vi "GetConfig.vi"() -> (3 "mail info out":T1)   [LabVIEW 2017]
uses:
  <vilib>/Utility/config.llb/Read Key (String).vi
  <vilib>/Utility/config.llb/Read Key (I32).vi
  <vilib>/Utility/config.llb/NI_LVConfig.lvlib
panel:
  in  "mail info":T1={"host"="smtp-mail.outlook.com", "port"=587, "username"="", "password"="", "From"="", "to"="", "subject"=""}
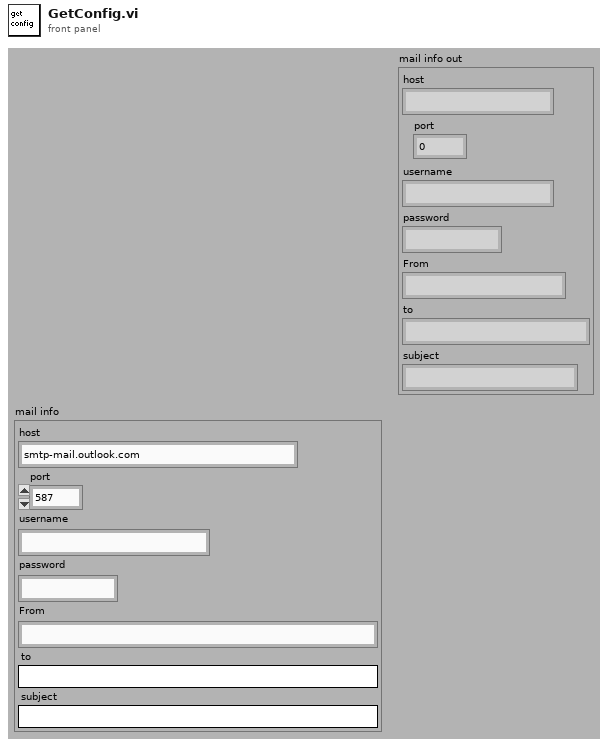
[diagram p1: front panel]
types:
  T1 = cluster{"host":string, "port":i32, "username":string, "password":string, "From":string, "to":string, "subject":string}
  T2 = enum32{"invalid app kind", "Development System", "Run Time System", "Student Edition", "Embedded LabVIEW", "Evaluation", "Custom"}
  T3 = typedef "NI_LVConfig.lvlib/Config Data RefNum.ctl" = refnum<k1>
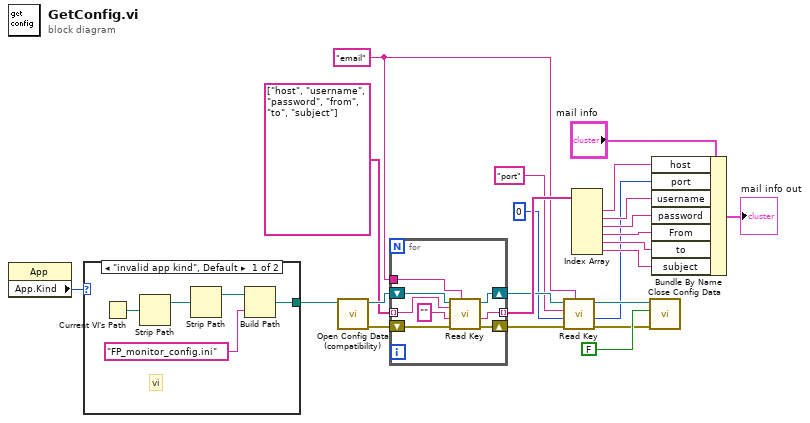
[diagram p0: block diagram]
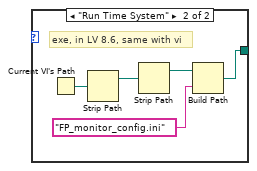
[diagram p2: hidden frame]
diagram:
  w5 = "email" ("key")
  n1 = property class="App"() -> ("App.Kind"=w2:T2)  [unwired: 2 in, 2 out]
  n2 = case shown="\"invalid app kind\", Default" w2 {
    tunnel: [w24 w30] -> w1
    frame "invalid app kind", Default {
      # "vi"
      n3 = Current VI's Path() -> (path=w28:path)
      n4 = Strip Path(path=w28) -> (stripped path=w27:path)  [unwired: 1 out]
      n5 = Strip Path(path=w27) -> (stripped path=w26:path)  [unwired: 1 out]
      n6 = Build Path(base path=w26, name or relative path="FP_monitor_config.ini" ("名称或相对路径")) -> (appended path=w24:path)
    }
    frame "Run Time System" {
      # "exe, in LV 8.6, same with vi"
      n7 = Current VI's Path() -> (path=w33:path)
      n8 = Strip Path(path=w33) -> (stripped path=w32:path)  [unwired: 1 out]
      n9 = Strip Path(path=w32) -> (stripped path=w29:path)  [unwired: 1 out]
      n10 = Build Path(base path=w29, name or relative path="FP_monitor_config.ini" ("名称或相对路径")) -> (appended path=w30:path)
    }
  }
  n11 = call <vilib>:"Open Config Data (compatibility).vi"("configuration file path"=w1) -> ("error out"=w21:errorcluster, "refnum"=w23:T3)  [unwired: 8 in, 1 out]
  n12 = for {
    shift-right: [w41] -> w9
    shift-left: w21 -> [w38]
    shift-right: [w37] -> w11
    shift-left: w23 -> [w40]
    tunnel: string[] ["host", "username", "password", "from", "to", "subject"] -> [w36] mode=indexing
    tunnel: [w35] -> w18 mode=indexing
    tunnel: w5 -> [w34]
    n13 = call-poly <vilib>:"Read Key.vi"("section"=w34, "error in (no error)"=w38, "default value"="" ("key"), "key"=w36, "refnum"=w40) -> ("error out"=w41:errorcluster, "value"=w35:string, "refnum out"=w37:T3)  [unwired: 1 in, 3 out]
  }
  n14 = call-poly <vilib>:"Read Key.vi"("section"=w5, "error in (no error)"=w9, "default value"=0 ("port"), "key"="port", "refnum"=w11) -> ("error out"=w8:errorcluster, "value"=w4:i32, "refnum out"=w10:T3)  [unwired: 4 out]
  n15 = Index Array(array=w18) -> (element #1=w17:string, element #2=w16:string, element #3=w15:string, element #4=w14:string, element #5=w13:string, element #6=w12:string)  [unwired: 6 in]
  n16 = call <vilib>:"Close Config Data.vi"("error in (no error)"=w8, "write file if changed (T)"=FALSE ("write configuration file? (T)"), "refnum"=w10) -> ()  [unwired: 9 out]
  n17 = Bundle By Name(cluster="mail info", "host"=w17, "port"=w4, "username"=w16, "password"=w15, "From"=w14, "to"=w13, "subject"=w12) -> (→"mail info out":T1)
